vi "SetCameraProperties.vi"() -> ()   [LabVIEW 2010]
uses:
  EDSDK-Labview.llb/kEdsProperties.ctl
panel:
  out "GetPropertyData":u8[](array[numeric]) format="%.0x"
  in  "SetPropertyData":u8[](array[numeric])=[2, 0, 0, 0] format="%.0x"
  in  "camera index":u32 min=1 max=1
  in  "stop":bool
  in  "SetPropertyID":T1=1280 items=["Unknown"=65535, "ProductName"=2, "BodyID"=3, "OwnerName"=4, "MakerName"=5, "DateTime"=6, "FirmwareVersion"=7, "BatteryLevel"=8, "CFn"=9, "SaveTo"=11, "CurrentStorage"=12, "CurrentFolder"=13, "MyMenu"=14, "BatteryQuality"=16, "HDDirectoryStructure"=32, "ImageQuality"=256, "JpegQuality"=257, "Orientation"=258, "ICCProfile"=259, "FocusInfo"=260, "DigitalExposure"=261, "WhiteBalance"=262, "ColorTemperature"=263, "WhiteBalanceShift"=264, "Contrast"=265, "ColorSaturation"=266, "ColorTone"=267, "Sharpness"=268, "ColorSpace"=269, "ToneCurve"=270, "PhotoEffect"=271, "FilterEffect"=272, "ToningEffect"=273, "ParameterSet"=274, "ColorMatrix"=275, "PictureStyle"=276, "PictureStyleDesc"=277, "ETTL2Mode"=279, "PictureStyleCaption"=512, "Linear"=768, "ClickWBPoint"=769, "WBCoeffs"=770, "GPSVersionID"=2048, "GPSLatitudeRef"=2049, "GPSLatitude"=2050, "GPSLongitudeRef"=2051, "GPSLongitude"=2052, "GPSAltitudeRef"=2053, "GPSAltitude"=2054, "GPSTimeStamp"=2055, "GPSSatellites"=2056, "GPSStatus"=2057, "GPSMapDatum"=2066, "GPSDateStamp"=2077, "AtCapture_Flag"=2147483648, "AEMode"=1024, "DriveMode"=1025, "ISOSpeed"=1026, "MeteringMode"=1027, "AFMode"=1028, "Av"=1029, "Tv"=1030, "ExposureCompensation"=1031, "FlashCompensation"=1032, "FocalLength"=1033, "AvailableShots"=1034, "Bracket"=1035, "WhiteBalanceBracket"=1036, "LensName"=1037, "AEBracket"=1038, "FEBracket"=1039, "ISOBracket"=1040, "NoiseReduction"=1041, "FlashOn"=1042, "RedEye"=1043, "FlashMode"=1044, "LensStatus"=1046, "Artist"=1048, "Copyright"=1049, "DepthOfField"=1051, "EFCompensation"=1054, "Evf_OutputDevice"=1280, "Evf_Mode"=1281, "Evf_WhiteBalance"=1282, "Evf_ColorTemperature"=1283, "Evf_DepthOfFieldPreview"=1284, "Evf_Zoom"=1287, "Evf_ZoomPosition"=1288, "Evf_FocusAid"=1289, "Evf_Histogram"=1290, "Evf_ImagePosition"=1291, "Evf_HistogramStatus"=1292, "Evf_AFMode"=1294, "Evf_CoordinateSystem"=1344, "Evf_ZoomRect"=1345]
  in  "SetParam":i32
  in  "GetParam":i32
  out "error out":errorcluster
  out "cameras":u32
  out "uint32":u32
  out "string":string
  in  "GetPropertyID":T1=1280 items=["Unknown"=65535, "ProductName"=2, "BodyID"=3, "OwnerName"=4, "MakerName"=5, "DateTime"=6, "FirmwareVersion"=7, "BatteryLevel"=8, "CFn"=9, "SaveTo"=11, "CurrentStorage"=12, "CurrentFolder"=13, "MyMenu"=14, "BatteryQuality"=16, "HDDirectoryStructure"=32, "ImageQuality"=256, "JpegQuality"=257, "Orientation"=258, "ICCProfile"=259, "FocusInfo"=260, "DigitalExposure"=261, "WhiteBalance"=262, "ColorTemperature"=263, "WhiteBalanceShift"=264, "Contrast"=265, "ColorSaturation"=266, "ColorTone"=267, "Sharpness"=268, "ColorSpace"=269, "ToneCurve"=270, "PhotoEffect"=271, "FilterEffect"=272, "ToningEffect"=273, "ParameterSet"=274, "ColorMatrix"=275, "PictureStyle"=276, "PictureStyleDesc"=277, "ETTL2Mode"=279, "PictureStyleCaption"=512, "Linear"=768, "ClickWBPoint"=769, "WBCoeffs"=770, "GPSVersionID"=2048, "GPSLatitudeRef"=2049, "GPSLatitude"=2050, "GPSLongitudeRef"=2051, "GPSLongitude"=2052, "GPSAltitudeRef"=2053, "GPSAltitude"=2054, "GPSTimeStamp"=2055, "GPSSatellites"=2056, "GPSStatus"=2057, "GPSMapDatum"=2066, "GPSDateStamp"=2077, "AtCapture_Flag"=2147483648, "AEMode"=1024, "DriveMode"=1025, "ISOSpeed"=1026, "MeteringMode"=1027, "AFMode"=1028, "Av"=1029, "Tv"=1030, "ExposureCompensation"=1031, "FlashCompensation"=1032, "FocalLength"=1033, "AvailableShots"=1034, "Bracket"=1035, "WhiteBalanceBracket"=1036, "LensName"=1037, "AEBracket"=1038, "FEBracket"=1039, "ISOBracket"=1040, "NoiseReduction"=1041, "FlashOn"=1042, "RedEye"=1043, "FlashMode"=1044, "LensStatus"=1046, "Artist"=1048, "Copyright"=1049, "DepthOfField"=1051, "EFCompensation"=1054, "Evf_OutputDevice"=1280, "Evf_Mode"=1281, "Evf_WhiteBalance"=1282, "Evf_ColorTemperature"=1283, "Evf_DepthOfFieldPreview"=1284, "Evf_Zoom"=1287, "Evf_ZoomPosition"=1288, "Evf_FocusAid"=1289, "Evf_Histogram"=1290, "Evf_ImagePosition"=1291, "Evf_HistogramStatus"=1292, "Evf_AFMode"=1294, "Evf_CoordinateSystem"=1344, "Evf_ZoomRect"=1345]
  # "LSB"
  # "MSB"
  # "LSB"
  # "MSB"
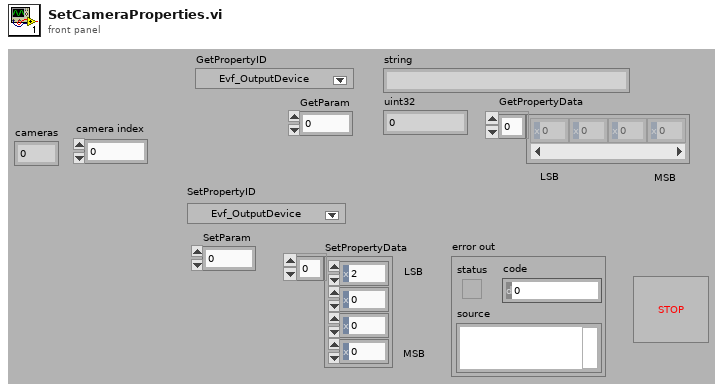
[diagram p1: front panel]
types:
  T1 = typedef "kEdsProperties.ctl" = u32
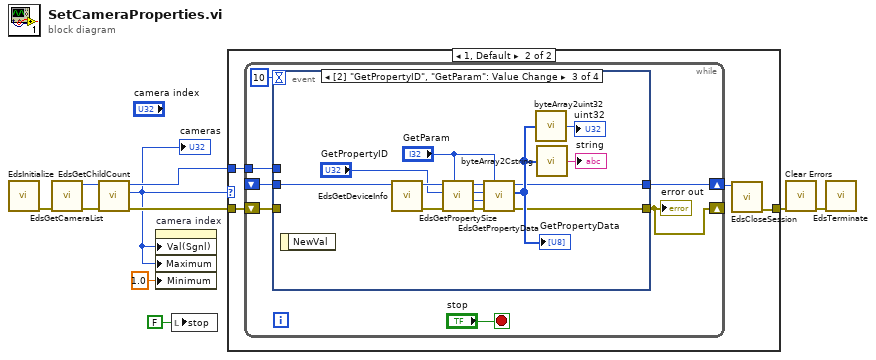
[diagram p0: block diagram]
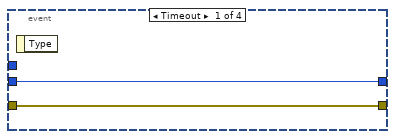
[diagram p3: hidden frame]
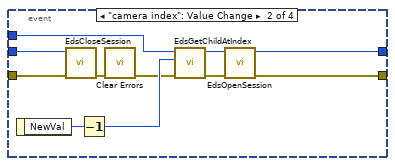
[diagram p4: hidden frame]
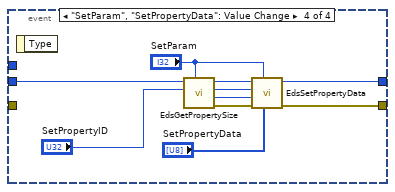
[diagram p5: hidden frame]
diagram:
  n1 = call "EdsInitialize.vi"() -> ("error out"=w10:errorcluster)  [unwired: 11 in]
  n2 = call "EdsGetCameraList.vi"("error in"=w10) -> ("error out"=w9:errorcluster, "outCameraListRef"=w7:u32)  [unwired: 9 in]
  n3 = call "EdsGetChildCount.vi"("error in"=w9, "inRef"=w7) -> ("error out"=w8:errorcluster, "count"=w3:u32, "inRef dup"=w6:u32)  [unwired: 7 in]
  "cameras" <- w3
  n4 = property on="camera index" class="DigNum (strict)"("Val(Sgnl)"=w3, "Maximum"=w3, "Minimum"=1.0 ("Data Entry Limits:Minimum")) -> ()  [unwired: 2 in, 2 out]
  n5 = local write "stop"(FALSE ("stop")) -> ()
  n6 = case shown="1, Default" w3 {
    tunnel: w8 -> [w11 w15]
    tunnel: w6 -> [_ w14]
    tunnel: [w11 w13] -> w2
    frame 0 {
    }
    frame 1, Default {
      n7 = while {
        tunnel: w14 -> [w21]
        shift-right: [w19] -> w12
        shift-left: _ -> [w18]
        shift-right: [w16] -> _
        shift-left: w15 -> [w22]
        stop <- "stop" stop-if-true
        n8 = event shown="[2] \"GetPropertyID\", \"GetParam\": Value Change" {
          selector: _ -> [_ _ _ _]
          dyn-events: _ -> [_ _ _ _]
          timeout: 10 -> [_ _ _ _]
          tunnel: w22 -> [w23 w25 _ _]
          tunnel: w21 -> [_ w29 _ _]
          tunnel: [w23 w28 w41 w52] -> w16
          tunnel: [w24 w31 w39 w50] -> w19
          tunnel: w18 -> [w24 w30 w40 w51]
          event Timeout {
            n9 = event-data() -> ()  [unwired: 1 in, 1 out]
          }
          event "camera index": Value Change {
            n10 = event-data() -> ("NewVal"=w33:u32)  [unwired: 1 in]
            n11 = call "EdsCloseSession.vi"("error in"=w25, "inCameraRef"=w30) -> ("error out"=w27:errorcluster)  [unwired: 8 in, 1 out]
            n12 = Decrement(x=w33) -> (x-1=w32:u32)
            n13 = call <vilib>:"Clear Errors.vi"("error in (no error)"=w27) -> ("error out"=w26:errorcluster)  [unwired: 6 in]
            n14 = call "EdsGetChildAtIndex.vi"("error in"=w26, "index"=w32, "inRef"=w29) -> ("error out"=w34:errorcluster, "outRef"=w35:u32)  [unwired: 7 in]
            n15 = call "EdsOpenSession.vi"("error in"=w34, "inCameraRef"=w35) -> ("error out"=w28:errorcluster, "inCameraRef dup"=w31:u32)  [unwired: 8 in]
          }
          event "GetParam": Value Change {
            n16 = event-data() -> ()  [unwired: 1 in, 1 out]
            n17 = call "EdsGetDeviceInfo.vi"("inCameraRef"=w40) -> ("error out"=w42:errorcluster, "inCameraRef dup"=w49:u32)  [unwired: 8 in, 1 out]
            n18 = call "EdsGetPropertySize.vi"("inParam"="GetParam", "error in"=w42, "inPropertyID"="GetPropertyID", "inRef"=w49) -> ("error out"=w37:errorcluster, "outSize"=w36:u32, "inPropertyID dup"=w44:T1, "inRef dup"=w48:u32)  [unwired: 3 in, 1 out]
            n19 = call "EdsGetPropertyData.vi"("inParam"="GetParam", "error in"=w37, "inPropertySize"=w36, "inPropertyID"=w44, "inRef"=w48) -> ("error out"=w41:errorcluster, "outPropertyData"=w45:u8[], "inRef dup"=w39:u32)  [unwired: 4 in]
            "GetPropertyData" <- w45
            n20 = call "byteArray2uint32.vi"("byteArray"=w45) -> ("uint32"=→"uint32":u32)
            n21 = call "byteArray2Cstring.vi"("byteArray"=w45) -> ("string"=→"string":string)
          }
          event "SetParam", "SetPropertyData": Value Change {
            n22 = event-data() -> ()  [unwired: 1 in, 1 out]
            n23 = call "EdsGetPropertySize.vi"("inParam"="SetParam", "inPropertyID"="SetPropertyID", "inRef"=w51) -> ("error out"=w58:errorcluster, "outSize"=w57:u32, "inPropertyID dup"=w54:T1, "inRef dup"=w59:u32)  [unwired: 4 in, 1 out]
            n24 = call "EdsSetPropertyData.vi"("inPropertyData"="SetPropertyData", "inParam"="SetParam", "error in"=w58, "inPropertySize"=w57, "inPropertyID"=w54, "inRef"=w59) -> ("error out"=w52:errorcluster, "inRef dup"=w50:u32)  [unwired: 4 in]
          }
        }
        "error out" <- w16
      }
      n25 = call "EdsCloseSession.vi"("inCameraRef"=w12) -> ("error out"=w13:errorcluster)  [unwired: 9 in, 1 out]
    }
  }
  n26 = call <vilib>:"Clear Errors.vi"("error in (no error)"=w2) -> ("error out"=w5:errorcluster)  [unwired: 6 in]
  n27 = call "EdsTerminate.vi"("error in"=w5) -> ()  [unwired: 10 in, 1 out]
